vi "Write Previous State Status.vi"(8 "error in (no error)":errorcluster, 10 "State Status":T1, 11 "Command States in":refnum<class "Command States.lvclass">) -> (0 "error out":errorcluster, 3 "Command States out":refnum<class "Command States.lvclass">)   [LabVIEW 2013, in "Command Actor.lvlib" / "Command States.lvclass"]
uses:
  Command States.lvclass
  Command/State Status.ctl
  Command States.lvclass/Command States.ctl
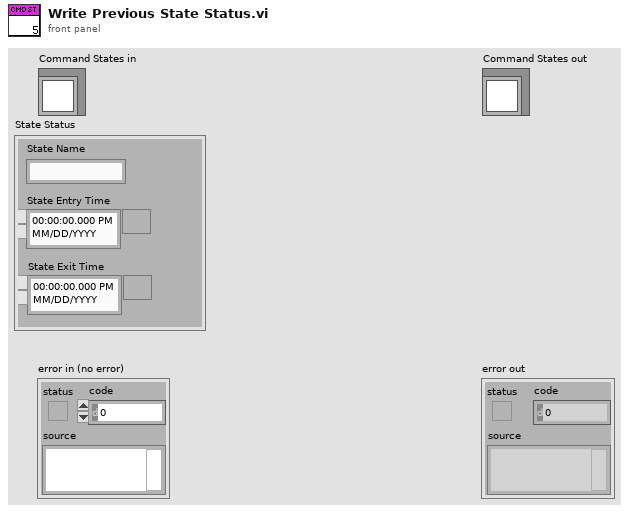
[diagram p1: front panel]
types:
  T1 = typedef "Command Actor.lvlib/Command States.lvclass/State Status.ctl" = cluster{"State Name":string, "State Entry Time":timestamp, "State Exit Time":timestamp}
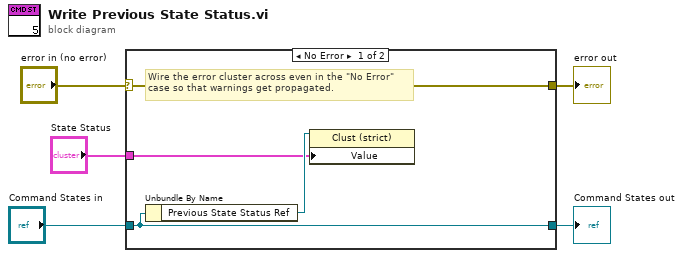
[diagram p0: block diagram]
diagram:
  n1 = case shown="No Error" "error in (no error)" {
    selector: "error in (no error)" -> [w9 w11]
    tunnel: [w9 w11] -> w4
    tunnel: [w8 w10] -> w2
    tunnel: "Command States in" -> [w8 w10]
    tunnel: "State Status" -> [w6 _]
    frame No Error {
      # "Wire the error cluster across even in the \"No Error\"\ncase so that warnings get propagated."
      n2 = Unbundle By Name(w8) -> ("Previous State Status Ref"=w7:refnum<vi>)
      n3 = property class="Clust (strict)"(reference=w7, "Value"=w6) -> ()  [unwired: 1 in, 2 out]
    }
    frame Error {
    }
  }
  "error out" <- w4
  "Command States out" <- w2
